vi "Acoustic THD Response.vi"(0 "TSM context":T1, 5 "Start dB SPL":dbl=94.0, 7 "End dB SPL":dbl=130.0, 9 "Delta dB SPL":dbl=1.0 format="%#_13g", 11 "Frequency":dbl=1000.0, 12 "Duration":dbl=2.0 format="%#_6p", 13 "Duration in Cycles? (F)":bool) -> (15 "error out":errorcluster)   [LabVIEW 2020]
doc: "Acoustic THD Response measure the THD of the DUT at various acoustic stimuli (dB SPL) with constant frequency and duration. Acoustic Functional Response Stepped Sine is used to get the THD (%) of the DUT."
uses:
  <vilib>/NI_TestStand_SemiconductorModule/NI_TestStand_Semiconductor_Module.lvlibp/PinMap/General/SemiconductorModuleContext.ctl
  Acoustic Frequency Response/Typedefs/Acoustic Sweep Config Cluster.ctl
  <vilib>/Analysis/1siggen.llb/Ramp Pattern.vi
  <vilib>/Analysis/1siggen.llb/Ramp Pattern by Delta.vi
  <vilib>/Utility/error.llb/Error Cluster From Error Code.vi
  <vilib>/NI_TestStand_SemiconductorModule/NI_TestStand_Semiconductor_Module.lvlibp
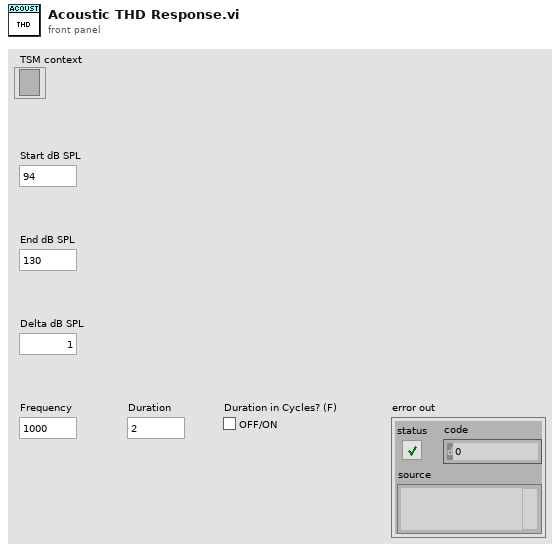
[diagram p1: front panel]
types:
  T1 = typedef "NI_TestStand_Semiconductor_Module.lvlibp/SemiconductorModuleContext.ctl" = refnum<k7>
  T2 = typedef "Acoustic Sweep Config Cluster.ctl" = cluster{"Frequency":dbl, "dB SPL":dbl, "Duration":dbl}
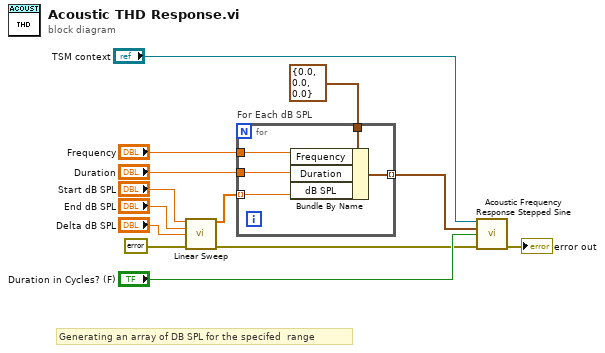
[diagram p0: block diagram]
diagram:
  # "Generating an array of DB SPL for the specifed  range"
  n1 = call "Linear Sweep.vi"("Start"="Start dB SPL", "End"="End dB SPL", "Delta"="Delta dB SPL", "error in (no error)"=errorcluster {"status"=FALSE, "code"=0, "source"=""}) -> ("Ramp Pattern"=w8:dbl[], "error out"=w3:errorcluster)  [unwired: 10 in]
  n2 = for "For Each dB SPL" {
    tunnel: T2 {"Frequency"=0.0, "dB SPL"=0.0, "Duration"=0.0} ("Cluster") -> [w18]
    tunnel: w8 -> [w17] mode=indexing
    tunnel: "Duration" -> [w16]
    tunnel: "Frequency" -> [w15]
    tunnel: [w14] -> w9 mode=indexing
    n3 = Bundle By Name(cluster=w18, "Frequency"=w15, "Duration"=w16, "dB SPL"=w17) -> (w14:T2)
  }
  n4 = call "Acoustic Frequency Response Stepped Sine.vi"("TSM context"="TSM context", "Sweep Configuration"=w9, "Duration in Cycles? (F)"="Duration in Cycles? (F)", "error in (no error)"=w3) -> ("error out"=→"error out":errorcluster)  [unwired: 11 in]
